vi "InstantiateNewAster.vi"(8 "error in":errorcluster, 11 "BaseAsteroidData":T1) -> (0 "error out":errorcluster, 3 "AsterRef":T3)   [LabVIEW 2017]
uses:
  ManRef_AsterData.ctl
  Asteroid/Asteroid_data.ctl
  GameConfig/GameConfig_data.ctl
  Asteroid/Asteroid_states.ctl
  HoldData/DataForColision.ctl
  HoldData/HoldData_mods.ctl
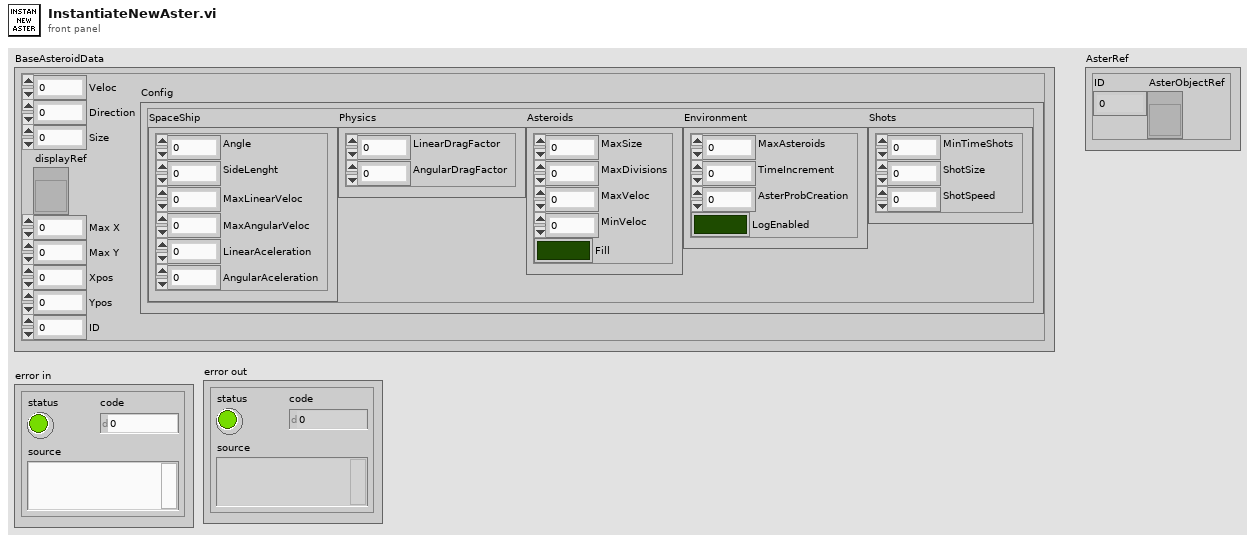
[diagram p1: front panel]
types:
  T1 = typedef "Asteroid_data.ctl" = cluster{"Veloc":dbl, "Direction":dbl, "Size":i32, "displayRef":refnum<vi>, "Max X":dbl, "Max Y":dbl, "Xpos":dbl, "Ypos":dbl, "ID":i32, "Config":T2}
  T2 = typedef "GameConfig_data.ctl" = cluster{"SpaceShip":cluster{"Angle":dbl, "SideLenght":dbl, "MaxLinearVeloc":dbl, "MaxAngularVeloc":dbl, "LinearAceleration":dbl, "AngularAceleration":dbl}, "Physics":cluster{"LinearDragFactor":dbl, "AngularDragFactor":dbl}, "Asteroids":cluster{"MaxSize":dbl, "MaxDivisions":i32, "MaxVeloc":dbl, "MinVeloc":dbl, "Fill":bool}, "Environment":cluster{"MaxAsteroids":i32, "TimeIncrement":dbl, "AsterProbCreation":dbl, "LogEnabled":bool}, "Shots":cluster{"MinTimeShots":dbl, "ShotSize":dbl, "ShotSpeed":dbl}}
  T3 = typedef "ManRef_AsterData.ctl" = cluster{"ID":i32, "AsterObjectRef":refnum<vi>}
  T4 = typedef "HoldData_mods.ctl" = enum16{"Init", "NewAster", "UpdateAster", "RemoveAster", "GetAsterData", "NewShoot", "UpdateShoot", "RemoveShoot", "GetShootData", "End"}
  T5 = typedef "DataForColision.ctl" = cluster{"X":dbl, "Y":dbl, "Size":dbl, "ID":i32}
  T6 = typedef "Asteroid_states.ctl" = enum16{"Init", "Move", "Split", "Draw", "Destroy"}
  T7 = typedef "LVBoundsTypeDef.ctl" = cluster{"Width":u32, "Height":u32}
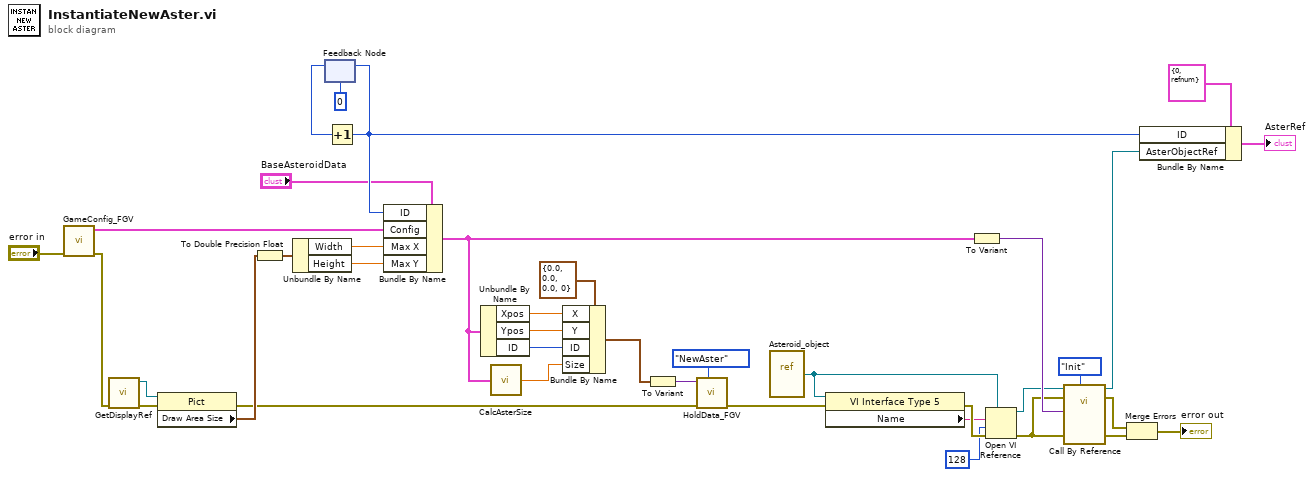
[diagram p0: block diagram]
diagram:
  n1 = call "GameConfig_FGV.vi"("error in"="error in") -> ("error out"=w33:errorcluster, "Config"=w12:T2)  [unwired: 9 in]
  n2 = call "GetDisplayRef.vi"("error in"=w33) -> ("error out"=w31:errorcluster, "Picture out"=w32:refnum<vi>)  [unwired: 9 in]
  n3 = property class="Pict"(reference=w32, error in=w31) -> (error out=w2:errorcluster, "Draw Area Size"=w35:T7)  [unwired: 1 out]
  n4 = To Double Precision Float(number=w35) -> (double precision float=w34:cluster{"Width":dbl, "Height":dbl})
  n5 = Unbundle By Name(w34) -> ("Width"=w37:dbl, "Height"=w38:dbl)
  n6 = feedback #1(0) -> (w15:i32)
  n7 = Increment(x=w15) -> (x+1=w36:i32)
  n8 = feedback-in #1(w36) -> ()
  n9 = Bundle By Name(cluster="BaseAsteroidData", "ID"=w36, "Config"=w12, "Max X"=w37, "Max Y"=w38) -> (w3:T1)
  n10 = Unbundle By Name(w3) -> ("Xpos"=w9:dbl, "Ypos"=w8:dbl, "ID"=w7:i32)
  n11 = call "CalcAsterSize.vi"("AsteroidData"=w3) -> ("AsteroidSize"=w10:dbl)
  n12 = Bundle By Name(cluster=T5 {"X"=0.0, "Y"=0.0, "Size"=0.0, "ID"=0} ("DataForColision"), "X"=w9, "Y"=w8, "ID"=w7, "Size"=w10) -> (w6:T5)
  n13 = To Variant(anything=w6) -> (Variant=w5:variant)
  n14 = call "HoldData_FGV.vi"("HoldData_mods"=HoldData_mods."NewAster", "error in"=w2, "DataIn"=w5) -> ("error out"=w1:errorcluster)  [unwired: 7 in, 1 out]
  n15 = vi-ref "Asteroid_object.vi"() -> (w29:refnum<vi>)
  n16 = property class="VI Interface Type 5"(reference=w29, error in=w1) -> (error out=w18:errorcluster, "Name"=w13:string)  [unwired: 1 out]
  n17 = To Variant(anything=w3) -> (Variant=w23:variant)
  n18 = Open VI Reference(type specifier VI Refnum (for type only)=w29, vi path=w13, options=128, error in (no error)=w18) -> (vi reference=w17:refnum<vi>, error out=w19:errorcluster)  [unwired: 2 in]
  n19 = call-by-ref "?"(reference=w17, error in=w19, "Asteroid_states"=Asteroid_states."Init", "error in"=w19, "DataIn"=w23) -> (reference out=w28:refnum<vi>, error out=w21:errorcluster, 0:"error out"=w20:errorcluster)  [unwired: 8 in]
  n20 = Merge Errors(w21, w20) -> (→"error out":errorcluster)
  n21 = Bundle By Name(cluster=T3 {"ID"=0, "AsterObjectRef"=refnum} ("DataCluster"), "ID"=w36, "AsterObjectRef"=w28) -> (→"AsterRef":T3)
